vi "Create Menu Folders for Folder Hierarchy.vi"(5 "Allow Initialization of AutoMenu on Target(T)":bool=TRUE, 7 "Refresh Palettes?(T)":bool=TRUE, 8 "error in (no error)":errorcluster, 9 "Force Auto Link?(F)":bool, 10 "Required Sub Folder for Menu Creation(.git)":string=".git", 11 "Target Main Folder":path=path "C:/Program Files (x86)/National Instruments/LabVIEW 2019/user.lib/_Tools") -> (0 "error out":errorcluster, 1 "Success?":bool=TRUE)   [LabVIEW 2019, in "AutoMenuCreator.lvlib"]
doc: "Folder hierarchy wrapper for 'Create Menu from Folder.vi'.\nFolders in the 'Target Main Folder' that contains the 'Required Sub Folder for Menu Creation' will be handled."
uses:
  AutoMenuCreator.lvlib
panel:
  in  "Stop":bool
  out "Progress":i32(slide) scale=0.0..10.0
  out "Active folder":string
  # "Progress"
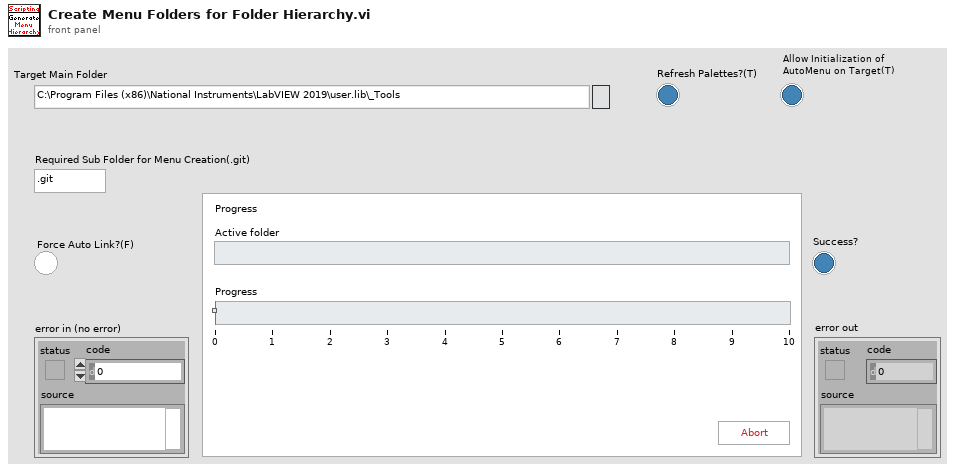
[diagram p1: front panel]
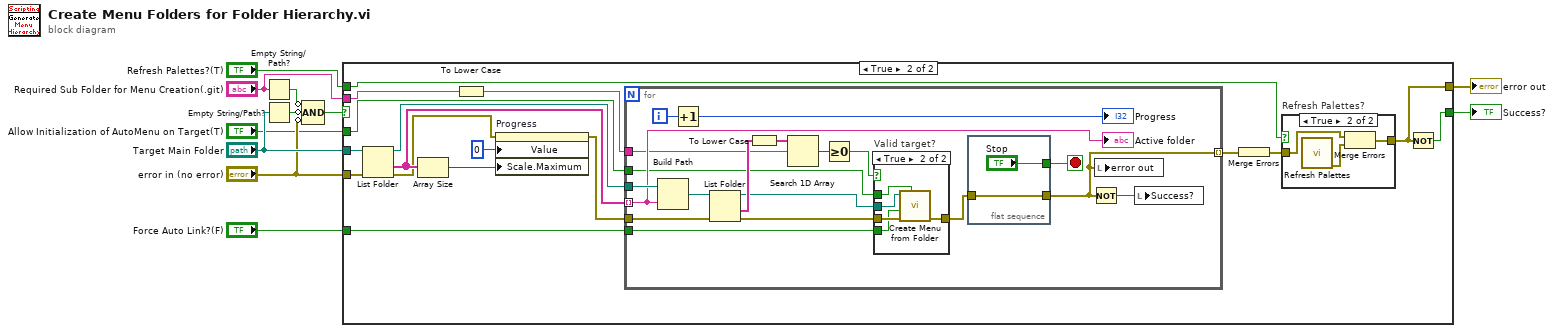
[diagram p0: block diagram]
diagram:
  n1 = Empty String/Path?(string/path="Required Sub Folder for Menu Creation(.git)") -> (empty?=w6:bool)
  n2 = Empty String/Path?(string/path="Target Main Folder") -> (empty?=w9:bool)
  n3 = Compound Arithmetic op=AND(invert w6, invert w9, invert "error in (no error)") -> (w7:bool)
  n4 = case shown="True" w7 {
    selector: w7 -> [w12 _]
    tunnel: "Target Main Folder" -> [_ w30]
    tunnel: [w13 w22] -> w11
    tunnel: "error in (no error)" -> [w13 w29]
    tunnel: [w12 w24] -> w5
    tunnel: "Required Sub Folder for Menu Creation(.git)" -> [_ w28]
    tunnel: "Refresh Palettes?(T)" -> [_ w21]
    tunnel: "Allow Initialization of AutoMenu on Target(T)" -> [_ w15]
    tunnel: "Force Auto Link?(F)" -> [_ w14]
    frame False {
    }
    frame True {
      n5 = List Folder(path=w30, error in=w29) -> (path out=w27:path, folder names=w20:string[], error out=w17:errorcluster)  [unwired: 2 in, 1 out]
      n6 = Array Size(array=w20) -> (size(s)=w19:i32)
      n7 = To Lower Case(string=w28) -> (all lower case string=w26:string)
      n8 = property on="Progress" class="Slide (strict)"(error in=w17, "Value"=0 ("Progress"), "Scale.Maximum"=w19) -> (error out=w16:errorcluster)  [unwired: 1 in, 1 out]
      n9 = for {
        tunnel: w26 -> [w48]
        tunnel: w20 -> [w52] mode=indexing
        tunnel: w27 -> [w53]
        tunnel: w16 -> [w46]
        tunnel: [w38] -> w25 mode=indexing
        tunnel: w15 -> [w36]
        tunnel: w14 -> [w35]
        i -> [w42]
        stop <- w40 stop-if-true
        n10 = Build Path(base path=w53, name or relative path=w52) -> (appended path=w51:path)
        n11 = Increment(x=w42) -> (x+1=→"Progress":i32)
        n12 = List Folder(path=w51, error in=w46) -> (path out=w43:path, folder names=w50:string[], error out=w44:errorcluster)  [unwired: 2 in, 1 out]
        n13 = To Lower Case(string=w50) -> (all lower case string=w49:string[])
        n14 = Search 1D Array(1D array=w49, element=w48) -> (index of element=w47:i32)  [unwired: 1 in]
        n15 = Greater Or Equal To 0?(x=w47) -> (x >= 0?=w45:bool)
        n16 = case "Valid target?" shown="True" w45 {
          tunnel: [w56 w59] -> w39
          tunnel: w44 -> [w56 w60]
          tunnel: w43 -> [_ w61]
          tunnel: w36 -> [_ w58]
          tunnel: w35 -> [_ w57]
          frame False {
          }
          frame True {
            n17 = call "Create Menu from Folder.vi"("Allow Initialization of AutoMenu on Target(T)"=w58, "error in (no error)"=w60, "Force Auto Link?(F)"=w57, "Target Folder"=w61) -> ("error out"=w59:errorcluster)  [unwired: 6 in, 1 out]
          }
        }
        n18 = flat-sequence {
          tunnel: ["Stop"] -> w40
          tunnel: [w54] -> w38
          tunnel: w39 -> [w54]
          frame #0 {
          }
        }
        n19 = Not(x=w38) -> (.not. x?=w37:bool)
        n20 = local write "error out"(w38) -> ()
        n21 = local write "Success?"(w37) -> ()
        "Active folder" <- w52
      }
      n22 = Merge Errors(w25) -> (w23:errorcluster)
      n23 = case "Refresh Palettes?" shown="True" w21 {
        tunnel: w23 -> [w31 w34]
        tunnel: [w31 w33] -> w22
        frame False {
        }
        frame True {
          n24 = call "Refresh Palettes.vi"() -> ("error out"=w32:errorcluster)  [unwired: 11 in]
          n25 = Merge Errors(w34, w32) -> (w33:errorcluster)
        }
      }
      n26 = Not(x=w22) -> (.not. x?=w24:bool)
    }
  }
  "error out" <- w11
  "Success?" <- w5
